vi "MovePattern.vi"(8 "error in (no error)":errorcluster, 10 "Project":string, 11 "Root In":path) -> (0 "error out":errorcluster, 3 "Root Out":path)   [LabVIEW 2019]
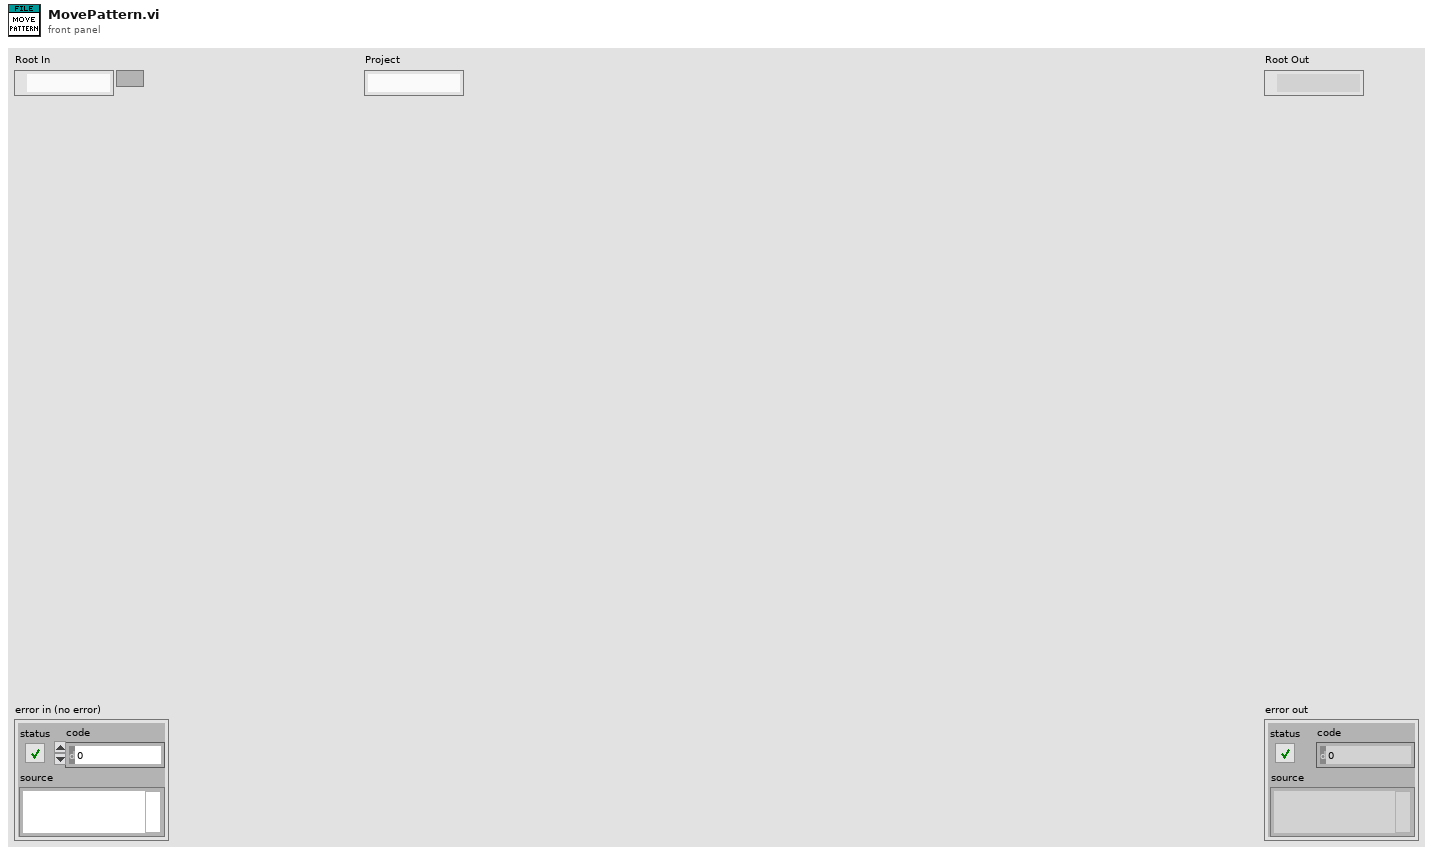
[diagram p1: front panel]
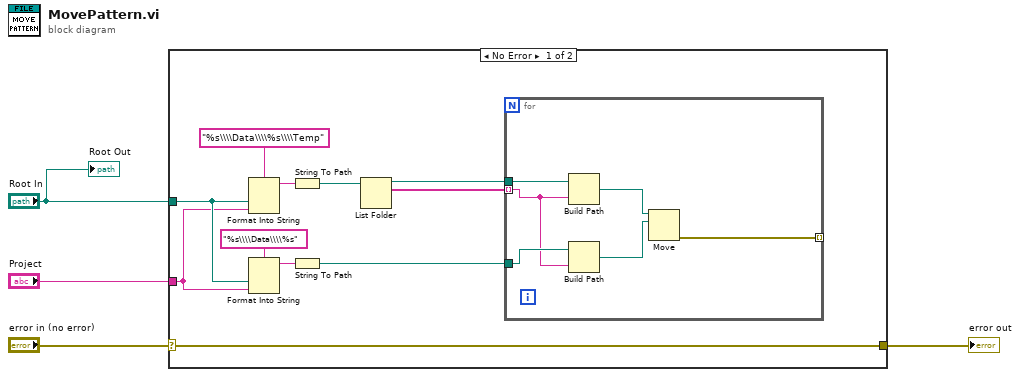
[diagram p0: block diagram]
diagram:
  n1 = case shown="No Error" "error in (no error)" {
    selector: "error in (no error)" -> [w13 w22]
    tunnel: "Root In" -> [w7 _]
    tunnel: [w13 w22] -> w2
    tunnel: "Project" -> [w6 _]
    frame No Error {
      n2 = Format Into String(format string="%s\\\\Data\\\\%s\\\\Temp", w7, w6) -> (resulting string=w14:string)  [unwired: 2 in, 1 out]
      n3 = Format Into String(format string="%s\\\\Data\\\\%s", w7, w6) -> (resulting string=w9:string)  [unwired: 2 in, 1 out]
      n4 = String To Path(string=w14) -> (path=w12:path)
      n5 = String To Path(string=w9) -> (path=w5:path)
      n6 = List Folder(path=w12) -> (path out=w11:path, filenames=w10:string[])  [unwired: 3 in, 2 out]
      n7 = for {
        tunnel: w11 -> [w21]
        tunnel: w10 -> [w18] mode=indexing
        tunnel: w5 -> [w19]
        tunnel: [w16] -> _ mode=indexing
        n8 = Build Path(base path=w21, name or relative path=w18) -> (appended path=w20:path)
        n9 = Build Path(base path=w19, name or relative path=w18) -> (appended path=w17:path)
        n10 = Move(source path=w20, 10:w17) -> (error out=w16:errorcluster)  [unwired: 3 in, 2 out]
      }
    }
    frame Error {
    }
  }
  "error out" <- w2
  "Root Out" <- "Root In"
